vi "string2datatype.vi"(11 "Ring Text.Text":string) -> (3 "datatype":T1(ring))   [LabVIEW 2014]
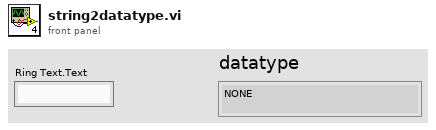
[diagram p1: front panel]
types:
  T1 = enum16{"NONE", "BINARY", "UNSIGNED_CHAR", "SIGNED_SHORT", "SIGNED_INT", "FLOAT", "COMPLEX", "DOUBLE", "RGB", "ALL"}
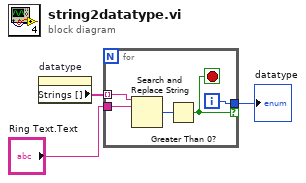
[diagram p0: block diagram]
diagram:
  n1 = property on="datatype" class="Enum (strict)"() -> ("Strings []"=w3:string[])  [unwired: 2 in, 2 out]
  n2 = for {
    tunnel: w3 -> [w7] mode=indexing
    tunnel: "Ring Text.Text" -> [w6]
    tunnel: [w8] -> w1 if=w4
    i -> [w8]
    stop <- w4 stop-if-true
    n3 = Search and Replace String(input string=w7, search string=w6) -> (number of replacements=w5:i32)  [unwired: 6 in, 3 out]
    n4 = Greater Than 0?(x=w5) -> (x > 0?=w4:bool)
  }
  "datatype" <- w1
